vi "Edit Read Register.vi"(8 "error in":errorcluster, 10 "TempController In":T1 caption="Read Register Data", 11 "Sequence Context In":refnum<k7>) -> (0 "error out":errorcluster, 2 "TempController Out":T1)   [LabVIEW 2023, in "LTT_TeststandSteptypes.lvlib"]
uses:
  LTT_TeststandSteptypes.lvlib
  HardwareAbstractionLayer_LVOOP/Modbus/Modbus_class/Teststand Steptypes/Control/ReadRegisterSteptypeControl.ctl
  HardwareAbstractionLayer_LVOOP/Database/SQL Public VI/Control/DB Options.ctl
  <vilib>/addons/TestStand/_TSUtility.llb/TestStand - Start Modal Dialog (Sequence Context).vi
  <vilib>/addons/TestStand/_TSUtility.llb/TestStand - End Modal Dialog (Sequence Context).vi
  HardwareAbstractionLayer_LVOOP/Database/Database.lvclass
  HardwareAbstractionLayer_LVOOP/Modbus/Modbus_class/Modbus.lvclass
panel:
  in  "Close":bool
  in  "OK":bool
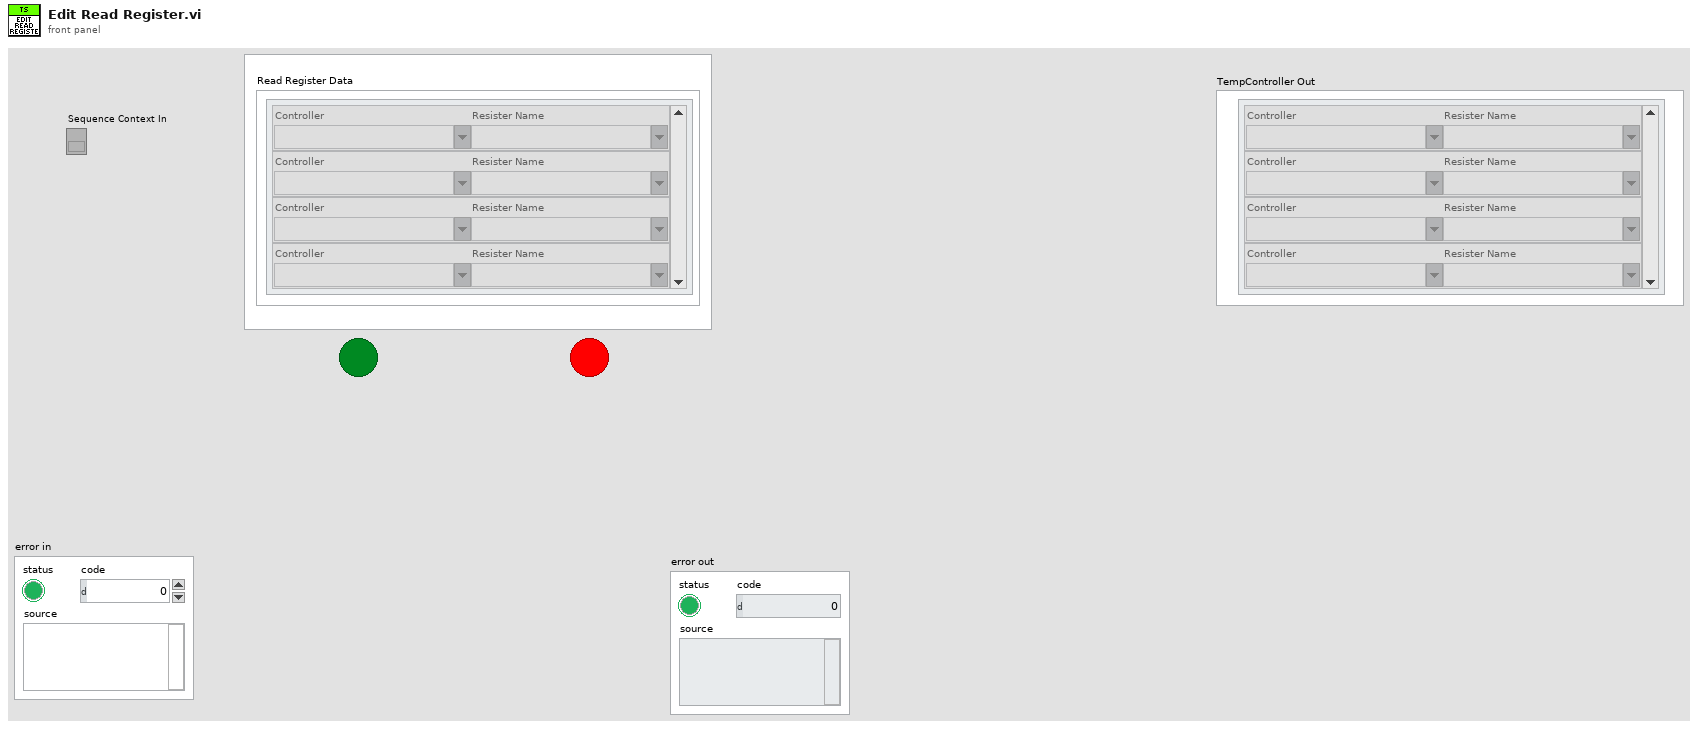
[diagram p1: front panel]
types:
  T1 = typedef "HardwareAbstractionLayer_LVOOP.lvlib/Modbus.lvclass/ReadRegisterSteptypeControl.ctl" = cluster{"Edit Controller":cluster{"Controller":string, "Resister Name":string}[]}
  T2 = typedef "HardwareAbstractionLayer_LVOOP.lvlib/Database.lvclass/DB Options.ctl" = enum16{"Init", "Select Data", "Insert Data", "Update Data", "Delete Data", "Execute Query", "Create Schema", "Create Table", "List Tables", "List Columns", "Close"}
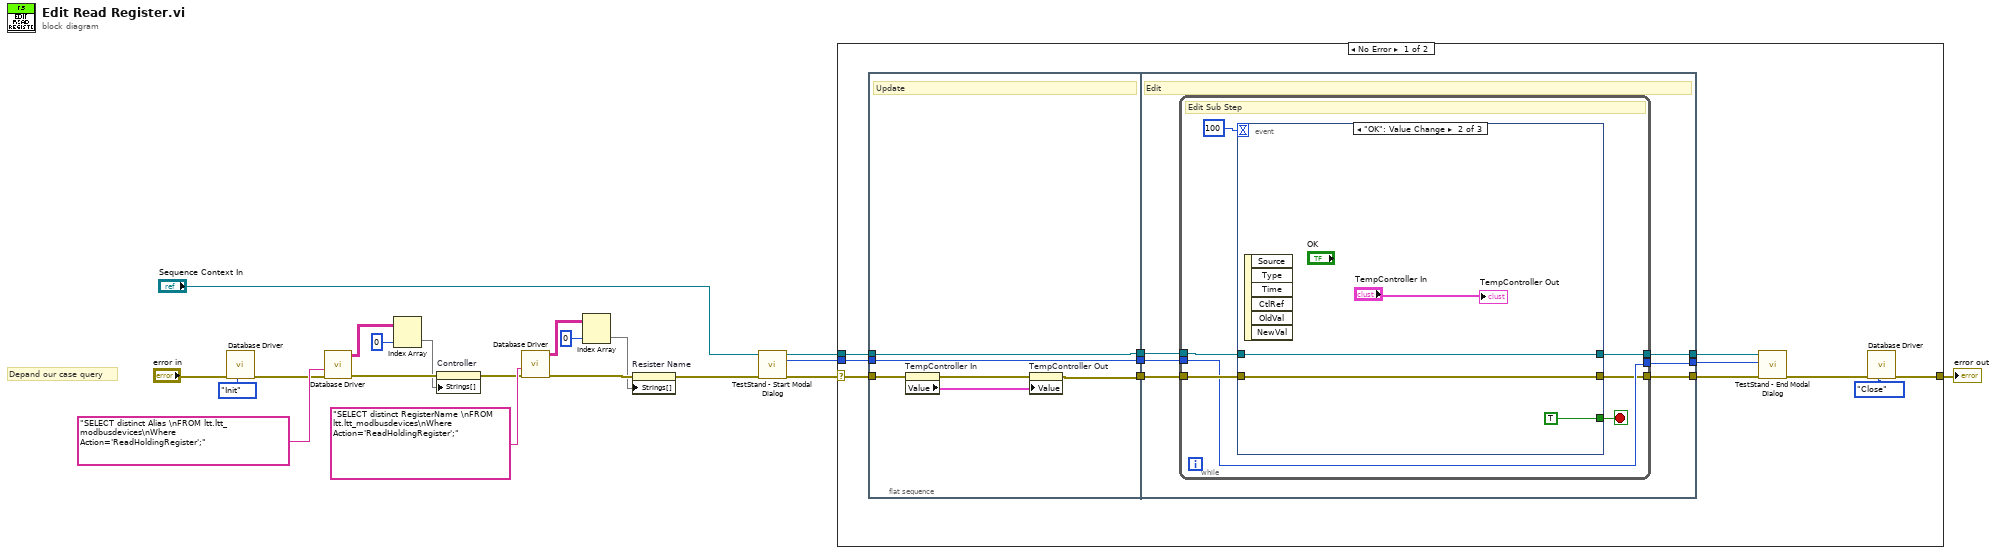
[diagram p0: block diagram]
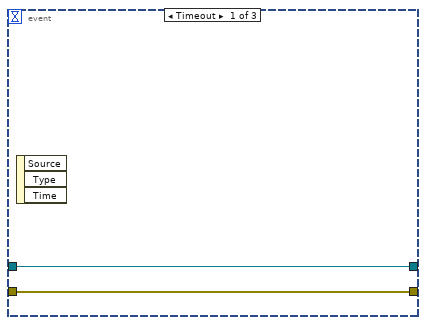
[diagram p2: hidden frame]
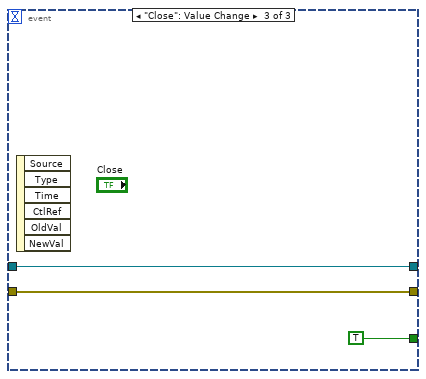
[diagram p3: hidden frame]
diagram:
  # "Depand our case query"
  n1 = call "Database Driver.vi"("Options"=DB_Options."Init", "error in"="error in") -> ("error out"=w13:errorcluster)  [unwired: 6 in, 3 out]
  n2 = call "Database Driver.vi"("error in"=w13, "SQL query"="SELECT distinct Alias \nFROM ltt.ltt_modbusdevices\nWhere Action='ReadHoldingRegister';") -> ("error out"=w6:errorcluster, "data"=w11:string[][])  [unwired: 6 in, 2 out]
  n3 = Index Array(array=w11, index (col)=0 ("index (row)")) -> (element=w5:string[])  [unwired: 1 in]
  n4 = property on="Controller" class="CmbBox"(error in=w6, "Strings[]"=w5) -> (error out=w4:errorcluster)  [unwired: 1 in, 1 out]
  n5 = call "Database Driver.vi"("error in"=w4, "SQL query"="SELECT distinct RegisterName \nFROM ltt.ltt_modbusdevices\nWhere Action='ReadHoldingRegister';") -> ("error out"=w3:errorcluster, "data"=w8:string[][])  [unwired: 6 in, 2 out]
  n6 = Index Array(array=w8, index (col)=0 ("index (row)")) -> (element=w1:string[])  [unwired: 1 in]
  n7 = property on="Resister Name" class="CmbBox"(error in=w3, "Strings[]"=w1) -> (error out=w2:errorcluster)  [unwired: 1 in, 1 out]
  n8 = call-poly <vilib>:"TestStand - Start Modal Dialog.vi"("Sequence Context In"="Sequence Context In", "error in (no error)"=w2) -> ("Sequence Context Out"=w17:refnum<k7>, "Modal ID"=w16:i32, "error out"=w18:errorcluster)  [unwired: 9 in, 2 out]
  n9 = case shown="No Error" w18 {
    selector: w18 -> [w29 w61]
    tunnel: w17 -> [w26 _]
    tunnel: w16 -> [w25 _]
    tunnel: [w22 w61] -> w14
    frame No Error {
      n10 = flat-sequence {
        tunnel: w29 -> [w36]
        tunnel: [w34] -> w32
        tunnel: w26 -> [w38]
        tunnel: w25 -> [w37]
        tunnel: [w38] -> w31
        tunnel: [w37] -> w30
        tunnel: w32 -> [w42]
        tunnel: [w40] -> w28
        tunnel: w31 -> [w44]
        tunnel: w30 -> [w43]
        tunnel: [w41] -> w24
        tunnel: [w39] -> w23
        frame #0 {
          # "Update"
          n11 = property on="TempController In" class="Clust (strict)"(error in=w36) -> (error out=w35:errorcluster, "Value"=w33:T1)  [unwired: 1 in, 1 out]
          n12 = property on="TempController Out" class="Clust (strict)"(error in=w35, "Value"=w33) -> (error out=w34:errorcluster)  [unwired: 1 in, 1 out]
        }
        frame #1 {
          # "Edit"
          n13 = while {
            tunnel: w44 -> [w49]
            tunnel: w43 -> [w46]
            tunnel: w42 -> [w47]
            tunnel: [w48] -> w39
            tunnel: [w46] -> w41
            tunnel: [w45] -> w40
            stop <- w50 stop-if-true
            # "Edit Sub Step"
            n14 = event shown="[1] \"OK\": Value Change" {
              selector: _ -> [_ _ _]
              dyn-events: _ -> [_ _ _]
              timeout: 100 -> [_ _ _]
              tunnel: [_ TRUE TRUE] -> w50
              tunnel: [w53 w56 w59] -> w48
              tunnel: w49 -> [w53 w56 w59]
              tunnel: w47 -> [w52 w55 w58]
              tunnel: [w52 w55 w58] -> w45
              event Timeout {
                n15 = event-data() -> ()  [unwired: 1 in, 3 out]
              }
              event "OK": Value Change {
                n16 = event-data() -> ()  [unwired: 1 in, 6 out]
                "TempController Out" <- "TempController In"
              }
              event "Close": Value Change {
                n17 = event-data() -> ()  [unwired: 1 in, 6 out]
              }
            }
          }
        }
      }
      n18 = call-poly <vilib>:"TestStand - End Modal Dialog.vi"("Sequence Context In"=w23, "Modal ID"=w24, "error in (no error)"=w28) -> ("error out"=w27:errorcluster)  [unwired: 12 in]
      n19 = call "Database Driver.vi"("Options"=DB_Options."Close", "error in"=w27) -> ("error out"=w22:errorcluster)  [unwired: 6 in, 3 out]
    }
    frame Error {
    }
  }
  "error out" <- w14
